vi "Read Nil.vi"   [LabVIEW 2017, in "LabPack.lvlib" / "Reader.lvclass"]
doc: "Reads and decodes a Nil value from the MessagePack data."
uses:
  Reader.lvclass
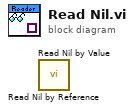
[diagram p0: block diagram]
diagram:
  n1 = call "Read Nil by Reference.vi"() -> ()  [unwired: 10 in, 2 out]
  n2 = call "Read Nil by Value.vi"() -> ()  [unwired: 10 in, 2 out]
